vi "Generate Signature.vi"(4 "consumer secret":string, 5 "Signature Method":T2=enum."HMAC-SHA1", 6 "token secret":string, 7 "HTTP Method":T3, 8 "error in (no error)":errorcluster, 10 "Parameters":T1[](array[typedef]), 11 "Base URL":string) -> (0 "error out":errorcluster, 2 "Signature":string)   [LabVIEW 2011, in "i3-oauth.lvlib"]
uses:
  i3-oauth.lvlib
  Controls/HTTP Method.ctl
  Controls/Signature Method.ctl
  Controls/key-value-pairs.ctl
panel:
  out "Signature Base string":string
  out "Parameter string":string
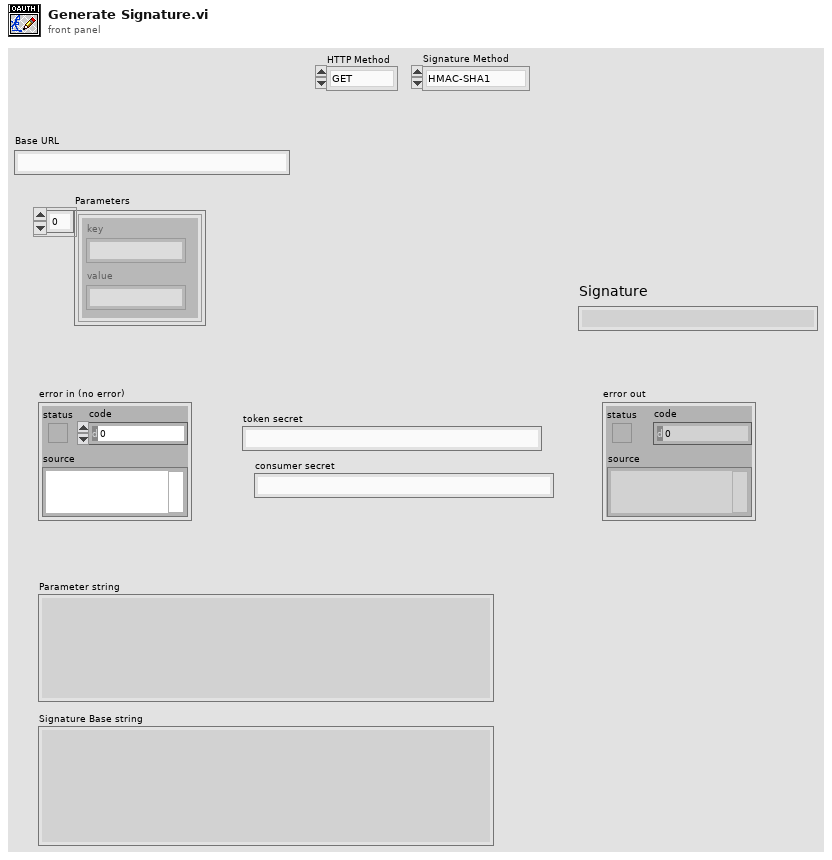
[diagram p1: front panel]
types:
  T1 = typedef "i3-oauth.lvlib/key-value-pairs.ctl" = cluster{"key":string, "value":string}
  T2 = typedef "i3-oauth.lvlib/Signature Method.ctl" = enum16{"HMAC-MD5", "HMAC-SHA1", "HMAC-SHA224", "HMAC-SHA256", "HMAC-SHA384", "HMAC-SHA512"}
  T3 = typedef "i3-oauth.lvlib/HTTP Method.ctl" = enum16{"GET", "POST", "PUT", "DELETE"}
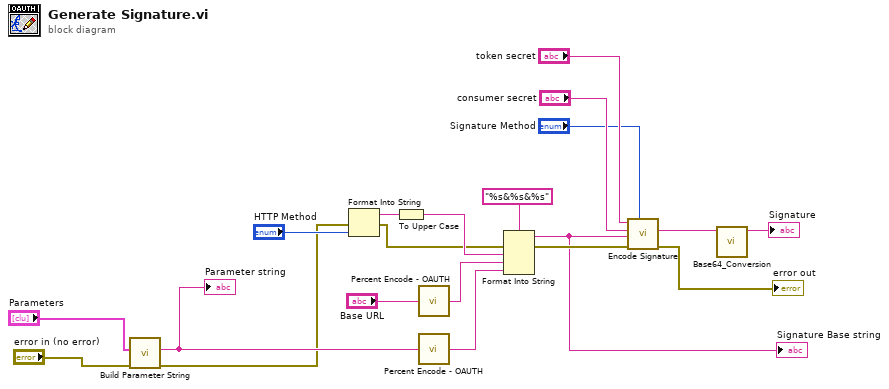
[diagram p0: block diagram]
diagram:
  n1 = call "Build Parameter String.vi"("error in (no error)"="error in (no error)", "Parameters"="Parameters") -> ("error out"=w2:errorcluster, "Parameter String"=w14:string)  [unwired: 8 in]
  "Parameter string" <- w14
  n2 = Format Into String(error in=w2, "HTTP Method") -> (resulting string=w8:string, error out=w3:errorcluster)  [unwired: 2 in]
  n3 = To Upper Case(1:w8) -> (0:w19:string)
  n4 = call "Percent Encode - OAUTH.vi"("unescaped string in"="Base URL") -> ("escaped string out"=w17:string)
  n5 = call "Percent Encode - OAUTH.vi"("unescaped string in"=w14) -> ("escaped string out"=w16:string)
  n6 = Format Into String(format string="%s&%s&%s", error in=w3, w19, w17, w16) -> (resulting string=w5:string, error out=w12:errorcluster)  [unwired: 1 in]
  "Signature Base string" <- w5
  n7 = call "Encode Signature.vi"("Signature Method"="Signature Method", "error in (no error)"=w12, "Signature Base string"=w5, "consumer secret"="consumer secret", "token secret"="token secret") -> ("error out"=→"error out":errorcluster, "Encoded Signature"=w11:string)  [unwired: 5 in]
  n8 = call "Base64_Conversion.vi"("String"=w11) -> ("Base64 String"=→"Signature":string)  [unwired: 10 in]
